vi "Log_PACKET - Add Packet to Queue_FORMAT.vi"(9 "Complete Packet":T1 {"Packet Data" format="%.0x"}) -> (2 "resulting string":string)   [LabVIEW 2014]
uses:
  PacketMode/SRV_PM_Packet.ctl
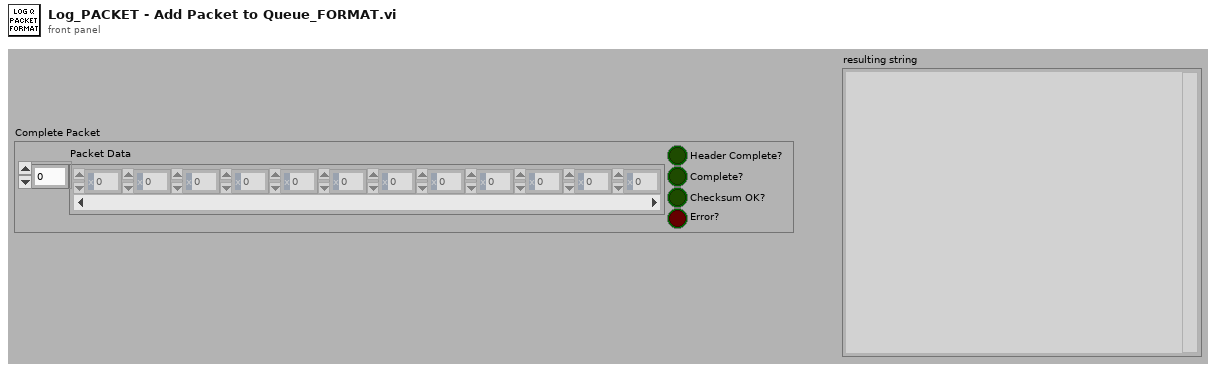
[diagram p1: front panel]
types:
  T1 = typedef "SRV_PM_Packet.ctl" = cluster{"Packet Data":u8[], "Header Complete?":bool, "Complete?":bool, "Checksum OK?":bool, "Error?":bool}
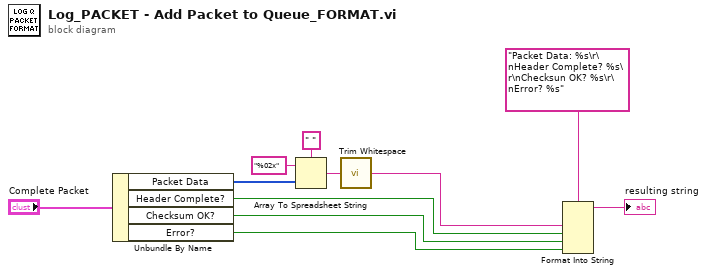
[diagram p0: block diagram]
diagram:
  n1 = Unbundle By Name("Complete Packet") -> ("Packet Data"=w8:u8[], "Header Complete?"=w4:bool, "Checksum OK?"=w3:bool, "Error?"=w2:bool)
  n2 = Array To Spreadsheet String(delimiter (Tab)=" ", array=w8, 3:"%02x" ("format string")) -> (spreadsheet string=w7:string)
  n3 = call <vilib>:"Trim Whitespace.vi"("string"=w7) -> ("trimmed string"=w5:string)  [unwired: 1 in]
  n4 = Format Into String(format string="Packet Data: %s\r\nHeader Complete? %s\r\nChecksun OK? %s\r\nError? %s", w5, w4, w3, w2) -> (resulting string=→"resulting string":string)  [unwired: 2 in, 1 out]
